vi "testa.vi"(4 "Enum":enum16{"keypad", "button"}(ring), 5 "Cluster":T2, 6 "volume":dbl=70.0) -> (1 "element":T1(ring), 2 "Boolean":bool=TRUE)   [LabVIEW 2014]
uses:
  <vilib>/sound2/lvsound2.llb/Sound Data Format.ctl
  <vilib>/sound2/lvsound2.llb/Sound Output Set Volume (Single).vi
  <vilib>/Utility/inputDevices.llb/keyboardAcquire.vi
  <vilib>/sound2/lvsound2.llb/Sound Output Write (DBL Single).vi
  <vilib>/Utility/inputDevices.llb/closeKeyboard.vi
  <vilib>/measure/NI_MABase.lvlib
panel:
  out "appended array":u32[](array[numeric])
  in  "stop":bool
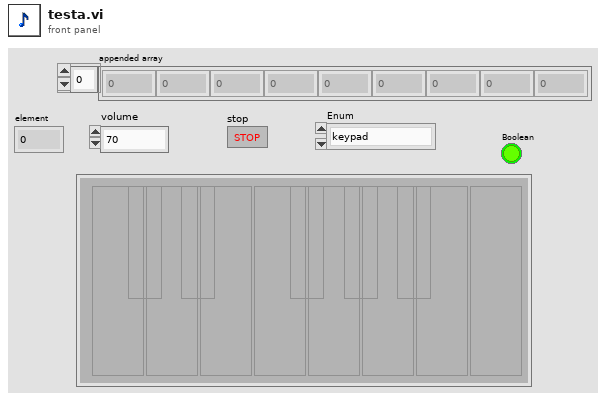
[diagram p1: front panel]
types:
  T1 = enum16{"0", "1", "2", "3", "4", "5", "6", "7", "8", "9", "A", "B", "C", "D", "E", "F", "G", "H", "I", "J", "K", "L", "M", "N", "O", "P", "Q", "R", "S", "T", "U", "V", "W", "X", "Y", "Z", "F1", "F2", "F3", "F4", "F5", "F6", "F7", "F8", "F9", "F10", "F11", "F12", "F13", "F14", "F15", "ADD", "BACK", "BACKSLASH", "CAPITAL", "COMMA", "DECIMAL", "DELETE", "DIVIDE", "DOWN", "END", "EQUALS", "ESCAPE", "GRAVE (`)", "HOME", "INSERT", "LBRACKET", "LCONTROL", "LEFT", "L ALT", "LSHIFT", "LWIN", "MINUS", "MULTIPLY", "NEXT", "NUMLOCK", "NUMPAD_0", "NUMPAD_1", "NUMPAD_2", "NUMPAD_3", "NUMPAD_4", "NUMPAD_5", "NUMPAD_6", "NUMPAD_7", "NUMPAD_8", "NUMPAD_9", "PAUSE", "PERIOD", "PRIOR (PG UP)", "RBRACKET", "RCONTROL", "RETURN", "RIGHT", "R ALT", "RSHIFT", "RWIN", "SCROLL", "SEMICOLON", "SLASH", "SPACE", "SUBTRACT", "TAB", "UP", "ENTER (num pad)", "' (quote)"}
  T2 = cluster{"c 2":bool, "c 3":bool, "c 4":bool, "c 5":bool, "c 6":bool, "c 7":bool, "c 8":bool, "c 9":bool, "c":bool, "c 10":bool, "c 11":bool, "c 12":bool, "c 13":bool}
  T3 = typedef "Sound Data Format.ctl" = cluster{"sample rate (S/s)":dbl, "number of channels":i32, "bits per sample":i32}
  T4 = typedef "Sound Output Task ID.ctl" = u32
  T5 = cluster{"sample rate (S/s)":dbl, "number of samples/ch":i32}
  T6 = enum16{"0", "1", "2", "3", "4", "5", "6", "7", "8", "9", "A", "B", "C", "D", "E", "F", "G", "H", "I", "J", "K", "L", "M", "N", "O", "P", "Q", "R", "S", "T", "U", "V", "W", "X", "Y", "Z", "F1", "F2", "F3", "F4", "F5", "F6", "F7", "F8", "F9", "F10", "F11", "F12", "F13", "F14", "F15", "ADD", "BACK", "BACKSLASH", "CAPITAL", "COMMA", "DECIMAL", "DELETE", "DIVIDE", "DOWN", "END", "EQUALS", "ESCAPE", "GRAVE (`)", "HOME", "INSERT", "LBRACKET", "LCONTROL", "LEFT", "L ALT", "LSHIFT", "LWIN", "MINUS", "MULTIPLY", "NEXT", "NUMLOCK", "NUMPAD_0", "NUMPAD_1", "NUMPAD_2", "NUMPAD_3", "NUMPAD_4", "NUMPAD_5", "NUMPAD_6", "NUMPAD_7", "NUMPAD_8", "NUMPAD_9", "PAUSE", "PERIOD", "PRIOR (PG UP)", "RBRACKET", "RCONTROL", "RETURN", "RIGHT", "R ALT", "RSHIFT", "RWIN", "SCROLL", "SEMICOLON", "SLASH", "SPACE", "SUBTRACT", "TAB", "UP", "ENTER (num pad)", "' (quote)"}[]
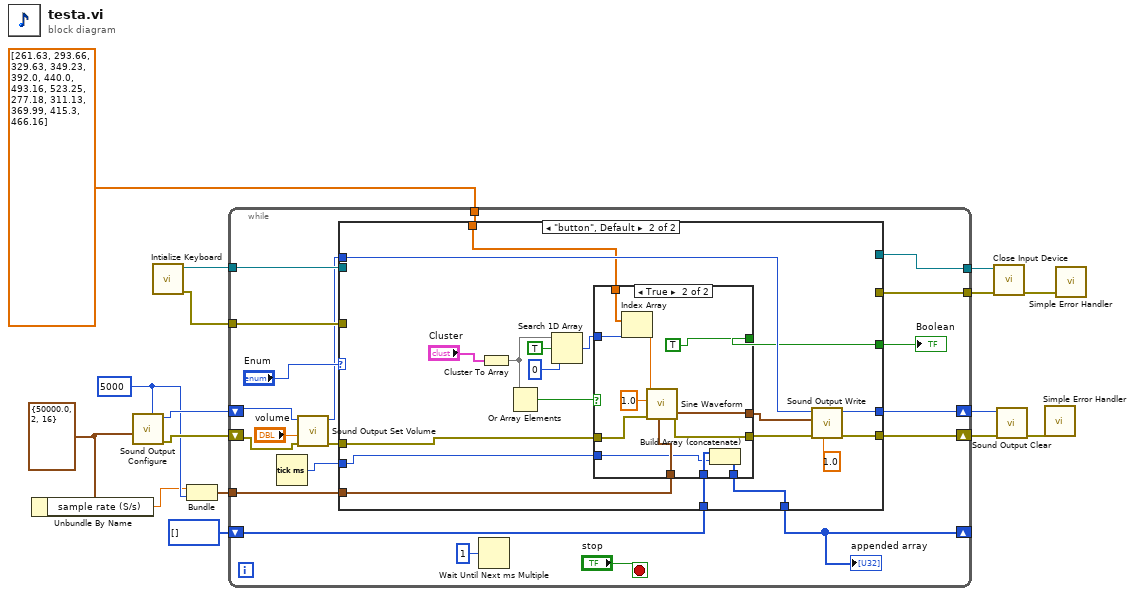
[diagram p0: block diagram]
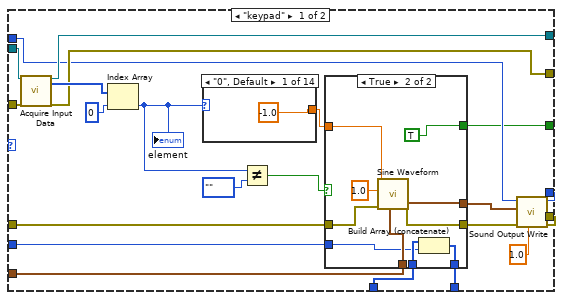
[diagram p2: hidden frame]
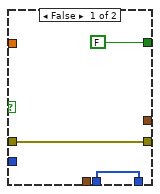
[diagram p3: hidden frame]
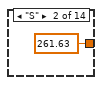
[diagram p4: hidden frame]
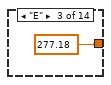
[diagram p5: hidden frame]
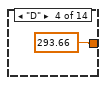
[diagram p6: hidden frame]
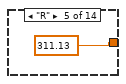
[diagram p7: hidden frame]
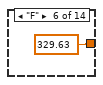
[diagram p8: hidden frame]
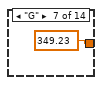
[diagram p9: hidden frame]
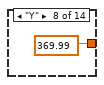
[diagram p10: hidden frame]
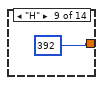
[diagram p11: hidden frame]
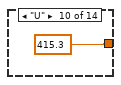
[diagram p12: hidden frame]
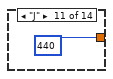
[diagram p13: hidden frame]
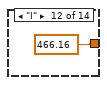
[diagram p14: hidden frame]
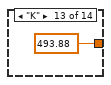
[diagram p15: hidden frame]
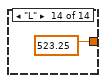
[diagram p16: hidden frame]
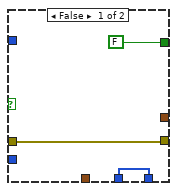
[diagram p17: hidden frame]
diagram:
  w13 = 5000 ("number of samples/ch")
  w14 = T3 {"sample rate (S/s)"=50000.0, "number of channels"=2, "bits per sample"=16} ("sound format")
  n1 = Unbundle By Name(w14) -> ("sample rate (S/s)"=w12:dbl)
  n2 = call <vilib>:"Sound Output Configure.vi"("number of samples/ch"=w13, "sound format"=w14) -> ("error out"=w15:errorcluster, "task ID"=w16:T4)  [unwired: 8 in]
  n3 = call <vilib>:"Intialize Keyboard.vi"() -> ("error out"=w5:errorcluster, "device ID"=w4:refnum<k1>)  [unwired: 10 in]
  n4 = Bundle("sample rate (S/s)"=w12, "number of samples/ch"=w13) -> (w11:T5)  [unwired: 1 in]
  n5 = while {
    tunnel: w11 -> [w33]
    tunnel: dbl[] [261.63, 293.66, 329.63, 349.23, 392.0, 440.0, 493.16, 523.25, 277.18, 311.13, 369.99, 415.3, 466.16] -> [w29]
    shift-right: [w32] -> w10
    shift-left: w16 -> [w35]
    shift-right: [w31] -> w9
    shift-left: w15 -> [w30]
    tunnel: w5 -> [w25]
    tunnel: w4 -> [w24]
    tunnel: [w23] -> w3
    tunnel: [w22] -> w2
    shift-right: [w18] -> _
    shift-left: u32[] [] -> [w19]
    stop <- "stop" stop-if-true
    n6 = Tick Count (ms)() -> (millisecond timer value=w17:u32)
    n7 = call-poly <vilib>:"Sound Output Set Volume.vi"("error in (no error)"=w30, "volume"="volume", "task ID"=w35) -> ("error out"=w34:errorcluster, "task ID out"=w21:T4)  [unwired: 7 in]
    n8 = case shown="\"button\", Default" "Enum" {
      tunnel: w34 -> [w45 w104]
      tunnel: w33 -> [w44 w101]
      tunnel: w21 -> [w43 w100]
      tunnel: [w42 w99] -> w32
      tunnel: [w41 w98] -> w31
      tunnel: w29 -> [_ w97]
      tunnel: w25 -> [w49 _]
      tunnel: w24 -> [w48 _]
      tunnel: [w47 _] -> w23
      tunnel: [w46 _] -> w22
      tunnel: [w40 w89] -> w20
      tunnel: w19 -> [w39 w88]
      tunnel: [w38 w87] -> w18
      tunnel: w17 -> [w37 w86]
      frame "keypad" {
        n9 = call-poly <vilib>:"Acquire Input Data.vi"("device ID"=w48, "error in (no error)"=w49) -> ("device ID"=w47:refnum<k1>, "keys pressed"=w54:T6, "error out"=w46:errorcluster)  [unwired: 15 in]
        n10 = Index Array(array=w54, index=0) -> (element=w58:T1)
        "element" <- w58
        n11 = case shown="\"0\", Default" w58 {
          tunnel: [-1.0 261.63 277.18 293.66 311.13 329.63 349.23 369.99 392 415.3 440 466.16 493.88 523.25] -> w53
          frame "0", Default {
          }
          frame "S" {
          }
          frame "E" {
          }
          frame "D" {
          }
          frame "R" {
          }
          frame "F" {
          }
          frame "G" {
          }
          frame "Y" {
          }
          frame "H" {
          }
          frame "U" {
          }
          frame "J" {
          }
          frame "I" {
          }
          frame "K" {
          }
          frame "L" {
          }
        }
        n12 = Not Equal?(x=w58, y=enum16{""}."") -> (x != y?=w57:bool)
        n13 = case shown="True" w57 {
          tunnel: w45 -> [w61 w70]
          tunnel: [_ w69] -> w50
          tunnel: [w61 w68] -> w51
          tunnel: w44 -> [_ w67]
          tunnel: w53 -> [_ w66]
          tunnel: [FALSE TRUE] -> w40
          tunnel: w39 -> [w59 w64]
          tunnel: [w59 w63] -> w38
          tunnel: w37 -> [_ w62]
          frame False {
          }
          frame True {
            n14 = call <vilib>:"Sine Waveform.vi"("sampling info"=w67, "error in (no error)"=w70, "amplitude"=1.0, "frequency"=w66) -> ("error out"=w68:errorcluster, "signal out"=w69:waveform(dbl))  [unwired: 6 in]
            n15 = Build Array (concatenate)(w64, w62) -> (w63:u32[])
          }
        }
        n16 = call-poly <vilib>:"Sound Output Write.vi"("timeout (sec)"=1.0, "error in (no error)"=w51, "data"=w50, "task ID"=w43) -> ("error out"=w41:errorcluster, "task ID out"=w42:T4)  [unwired: 6 in]
      }
      frame "button", Default {
        n17 = Cluster To Array(cluster="Cluster") -> (array=w92:bool[])
        n18 = Or Array Elements(Boolean array=w92) -> (logical OR=w91:bool)
        n19 = Search 1D Array(1D array=w92, element=TRUE, start index (0)=0) -> (index of element=w90:i32)
        n20 = case shown="True" w91 {
          tunnel: w104 -> [w107 w118]
          tunnel: [_ w117] -> w103
          tunnel: [w107 w116] -> w102
          tunnel: w101 -> [_ w115]
          tunnel: w97 -> [_ w114]
          tunnel: w90 -> [_ w113]
          tunnel: [FALSE TRUE] -> w89
          tunnel: w88 -> [w105 w110]
          tunnel: [w105 w109] -> w87
          tunnel: w86 -> [_ w108]
          frame False {
          }
          frame True {
            n21 = Index Array(array=w114, index=w113) -> (element=w112:dbl)
            n22 = call <vilib>:"Sine Waveform.vi"("sampling info"=w115, "error in (no error)"=w118, "amplitude"=1.0, "frequency"=w112) -> ("error out"=w116:errorcluster, "signal out"=w117:waveform(dbl))  [unwired: 6 in]
            n23 = Build Array (concatenate)(w110, w108) -> (w109:u32[])
          }
        }
        n24 = call-poly <vilib>:"Sound Output Write.vi"("timeout (sec)"=1.0, "error in (no error)"=w102, "data"=w103, "task ID"=w100) -> ("error out"=w98:errorcluster, "task ID out"=w99:T4)  [unwired: 6 in]
      }
    }
    "Boolean" <- w20
    "appended array" <- w18
    n25 = Wait Until Next ms Multiple(millisecond multiple=u32 1) -> ()  [unwired: 1 out]
  }
  n26 = call-poly <vilib>:"Close Input Device.vi"("error in (no error)"=w2, "device ID"=w3) -> ("error out"=w6:errorcluster)  [unwired: 8 in]
  n27 = call <vilib>:"Sound Output Clear.vi"("error in (no error)"=w9, "task ID"=w10) -> ("error out"=w8:errorcluster)  [unwired: 9 in]
  n28 = call <vilib>:"Simple Error Handler.vi"("error in (no error)"=w8) -> ()  [unwired: 4 in, 5 out]
  n29 = call <vilib>:"Simple Error Handler.vi"("error in (no error)"=w6) -> ()  [unwired: 4 in, 5 out]
